vi "SC TCP Unflatten Response.vi"(8 "error in":errorcluster, 11 "Response JSON":string) -> (0 "error out":errorcluster, 3 "Response Details":T1)   [LabVIEW 2018]
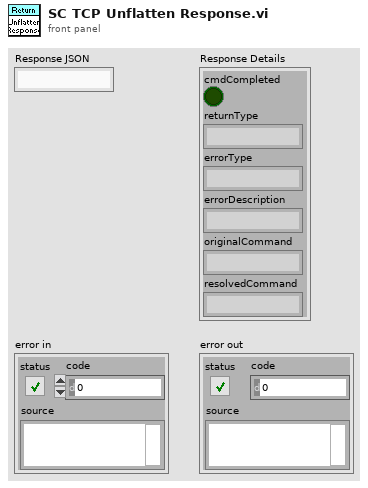
[diagram p1: front panel]
types:
  T1 = cluster{"cmdCompleted":bool, "returnType":string, "errorType":string, "errorDescription":string, "originalCommand":string, "resolvedCommand":string}
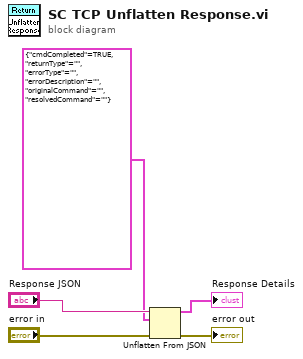
[diagram p0: block diagram]
diagram:
  n1 = Unflatten From JSON(JSON string="Response JSON", type and defaults=T1 {"cmdCompleted"=TRUE, "returnType"="", "errorType"="", "errorDescription"="", "originalCommand"="", "resolvedCommand"=""}, error in (no error)="error in") -> (value=→"Response Details":T1, error out=→"error out":errorcluster)  [unwired: 4 in]
